vi "FixArray.vi"(1 "PreviousState":dbl[][](array[numeric]), 2 "Cluster":cluster{"Numeric":dbl, "Numeric 2":dbl}, 3 "Array 3":dbl[](array[numeric])) -> (0 "NewState":dbl[][](array[numeric]))   [LabVIEW 2014]
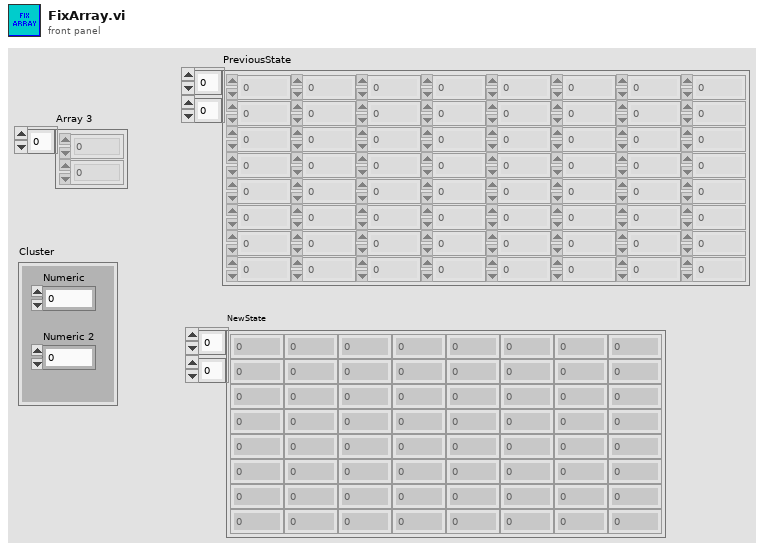
[diagram p1: front panel]
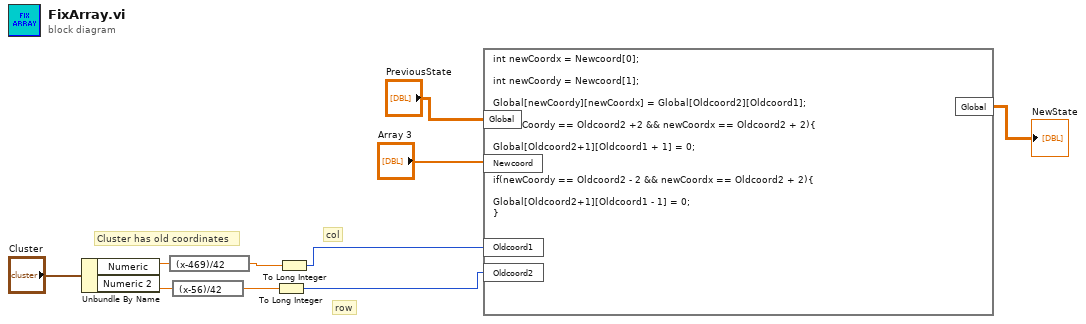
[diagram p0: block diagram]
diagram:
  # "row"
  # "col"
  # "Cluster has old coordinates"
  n1 = Unbundle By Name("Cluster") -> ("Numeric"=w9:dbl, "Numeric 2"=w7:dbl)
  n2 = expression code="(x-469)/42"(w9) -> (w10:dbl)
  n3 = expression code="(x-56)/42"(w7) -> (w8:dbl)
  n4 = To Long Integer(number=w8) -> (32bit integer=w2:i32)
  n5 = To Long Integer(number=w10) -> (32bit integer=w3:i32)
  n6 = formula code="int newCoordx = Newcoord[0];\n\nint newCoordy = Newcoord[1];\n\nGlobal[newCoordy][newCoordx] = Global[Oldcoord2][Oldcoord1];\n\nif(newCoordy == Oldcoord2 +2 && newCoordx == Oldcoord2 + 2){\n\nGlobal[Oldcoord2+1][Oldcoord1 + 1] = 0;\n}\n\nif(newCoordy == Oldcoord2 - 2 && newCoordx == Oldcoord2 + 2){\n\nGlobal[Oldcoord2+1][Oldcoord1 - 1] = 0;\n}"("Global"="PreviousState", "Newcoord"="Array 3", "Oldcoord1"=w3, "Oldcoord2"=w2) -> ("Global"=→"NewState":dbl[][])
